vi "_VEL.vi"(0 "System no.":i32=1 min=1 max=4 step=1, 2 "Axes to set":string[](array[string]), 3 "Velocity values":dbl[](array[numeric]) format="%.6f", 4 "No.of digits":i16=4, 5 "error in":errorcluster, 6 "Without axis ID?":bool) -> (14 "Controller error":bool, 19 "error out":errorcluster)   [LabVIEW 2015]
doc: "Sets velocity and checks for error. If Without axis ID? is TRUE, then Axes to set is ignored and first field of Velocity values array is used for velocity command. The velocity should not be set to 0. Number of digits is the number of digits after the decimal point in the velocity value(s) that will be sent. Controller error is TRUE if selected system reports an error code which is not 0.\n\nValid for Analog systems, C-702, C-843, C-843.PM, C-844, C-848, C-865, C-866, C-867, C-880, C-880K005, E-516, E-517, E-710, E-712, E-725, E-753, E-755, E-761, E-861, F-206, M-8X0, Mercury™. To support analog interfacing, VI must be present for E-816 also.\n\nAnalog: Without axis ID? = FALSE; Velocity unit is µm/sec\n\nC-867: Without axis ID? = FALSE. Velocity unit is mm/s. The VEL command saves the parameters in RAM only. To save the currently valid parameters to flash ROM, where they become the power-on defaults, you must run WPA.vi. Parameter changes not saved with WPA will be lost when the C-867 is powered off.\n\nC-880: Without axis ID? = FALSE, for NanoCube axes command is not valid\n\nC-880K005: VI only supported when called through PI_Multix.vi\n\nE-516: Without axis ID? = FALSE. Velocity unit is µm/s. The VEL command saves the parameters in RAM only. To save the currently valid parameters to flash ROM, where they become the power-on defaults, you must run WPA.vi. Parameter changes not saved with WPA will be lost when the E-516 is powered off.\n\nE-517: Without axis ID? = FALSE. Velocity unit is µm/s in closed-loop operation and V/s in open-loop operation. Velocity settings made with VEL are present in RAM only and will be reset to default (\"Servo Loop Slew Rate\" value) when the controller is powered down or rebooted.\n\nE-712, E-725, E-753, E-861: Without axis ID? = FALSE. Velocity unit is µm/s. Velocity settings made with VEL are present in RAM only and will be reset to default (\"Servo Loop Slew Rate\" value) when the controller is powered down or rebooted.\n\nE-710: Without axis ID? = FALSE. Velocity unit is µm/ms.\n\nE-755: Without axis ID? = FALSE. Velocity unit is µm/s. Command not available for E-755.101.\n\nE-761: Without axis ID? = FALSE. Velocity unit is µm/ms.The VEL command saves the \"Servo Loop Slew Rate\" parameter in RAM only. To save the currently valid parameter to flash ROM, where it becomes the power-on defaults, you must run WPA.vi. Parameter changes not saved with WPA will be lost when the PC is powered off or the E-761 is rebooted.\n\nE-861: Without axis ID? = FALSE. The VEL setting only takes effect when the given axis is in closed-loop operation (servo on). For open-loop operation, use OVL instead. The maximum value which can be set with the VEL command is given by the Closed-loop velocity parameter, ID 0xA (can be changed with SPA and SEP). On power-on, the current closed-loop velocity is half the maximum.\n\nF-206: F-206 platform velocity: Without axis ID? = TRUE; velocity of axes A and/or B: Without axis ID? = False; axes K,L,M: command not valid\n\nM-8X0: M-8X0 platform velocity: Without axis ID? = TRUE; velocity of axes A and/or B: Without axis ID? = False\n\nAll other systems: Without axis ID? = FALSE"
panel:
  # "Sets velocity and checks for error.  If \"Without axis ID\" is TRUE, \nthen \"Axes to set\" is ignored and first field of \"Velocity values\" \narray is used for velocity command."
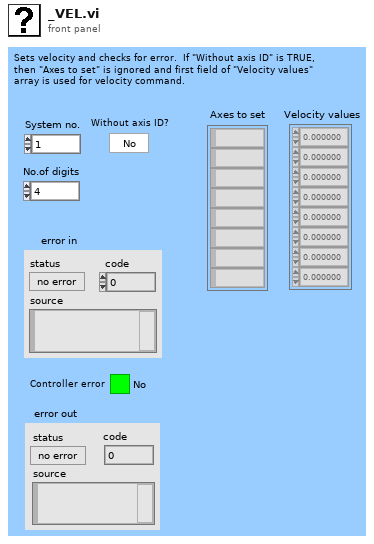
[diagram p1: front panel]
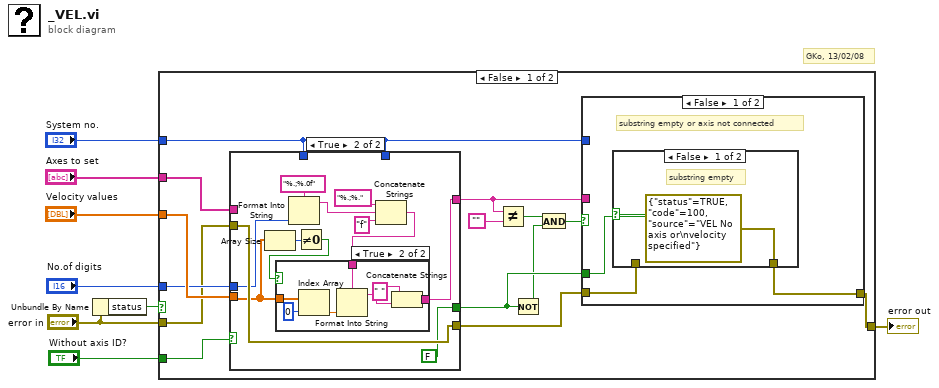
[diagram p0: block diagram]
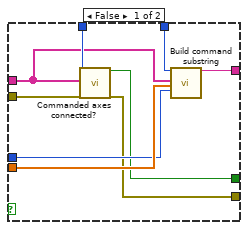
[diagram p2: hidden frame]
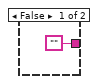
[diagram p3: hidden frame]
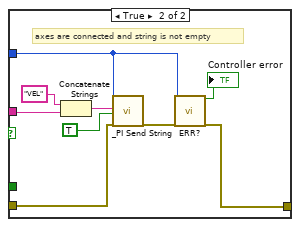
[diagram p5: hidden frame]
diagram:
  # "GKo, 13/02/08"
  n1 = Unbundle By Name("error in") -> ("status"=w2:bool)
  n2 = case shown="False" w2 {
    tunnel: [w22 w66] -> w8
    tunnel: "Velocity values" -> [w19 _]
    tunnel: "No.of digits" -> [w18 _]
    tunnel: "error in" -> [w17 w66]
    tunnel: "System no." -> [w9 _]
    tunnel: "Axes to set" -> [w15 _]
    tunnel: "Without axis ID?" -> [w10 _]
    frame False {
      n3 = case shown="True" w10 {
        tunnel: [w31 w41] -> w20
        tunnel: w19 -> [w30 w34]
        tunnel: w18 -> [w29 w36]
        tunnel: w17 -> [w28 w43]
        tunnel: [w27 w43] -> w16
        tunnel: w9 -> [w26 _]
        tunnel: w15 -> [w25 _]
        tunnel: [w24 FALSE] -> w13
        tunnel: w9 -> [w23 _]
        frame False {
          n4 = call "Commanded axes connected?.vi"("System no."=w26, "Commanded axes"=w25, "error in"=w28) -> ("Controller error"=w24:bool, "error out"=w27:errorcluster)  [unwired: 15 in]
          n5 = call "Build command substring.vi"("System no."=w23, "Affected axes"=w25, "Parameters"=w30, "No. of digits"=w29) -> ("Command substring"=w31:string)  [unwired: 15 in]
        }
        frame True {
          n6 = Array Size(array=w34) -> (size(s)=w33:i32)
          n7 = Format Into String(format string="%.;%.0f" ("Format String"), w36) -> (resulting string=w37:string)  [unwired: 2 in, 1 out]
          n8 = Not Equal To 0?(x=w33) -> (x != 0?=w32:bool)
          n9 = Concatenate Strings("%.;%." ("Format String"), w37, "f" ("Format String")) -> (w35:string)
          n10 = case shown="True" w32 {
            tunnel: ["" w47] -> w41
            tunnel: w35 -> [_ w46]
            tunnel: w34 -> [_ w45]
            frame False {
            }
            frame True {
              n11 = Index Array(array=w45, index=0 ("Index")) -> (element=w50:dbl)
              n12 = Format Into String(format string=w46, w50) -> (resulting string=w49:string)  [unwired: 2 in, 1 out]
              n13 = Concatenate Strings(" ", w49) -> (w47:string)
            }
          }
        }
      }
      n14 = Not Equal?(x=w20, y="") -> (x != y?=w14:bool)
      n15 = Not(x=w13) -> (.not. x?=w12:bool)
      n16 = And(x=w14, y=w12) -> (x .and. y?=w11:bool)
      n17 = case shown="False" w11 {
        tunnel: w20 -> [_ w64]
        tunnel: [w54 w59] -> w22
        tunnel: w16 -> [w52 w61]
        tunnel: w13 -> [w53 _]
        tunnel: w9 -> [_ w58]
        frame False {
          # "substring empty or axis not connected"
          n18 = case shown="False" w53 {
            tunnel: [errorcluster {"status"=TRUE, "code"=100, "source"="VEL No axis or\nvelocity specified"} ("error out") w56] -> w54
            tunnel: w52 -> [_ w56]
            frame False {
              # "substring empty"
            }
            frame True {
              # "commanded axis not connected"
            }
          }
        }
        frame True {
          # "axes are connected and string is not empty"
          n19 = Concatenate Strings("VEL", w64) -> (w62:string)
          n20 = call "_PI Send String.vi"("System no."=w58, "String to send"=w62, "Attach termination char.?"=TRUE ("Attach Linefeed?"), "error in"=w61) -> ("error out"=w60:errorcluster)  [unwired: 15 in]
          n21 = call "ERR?.vi"("System no."=w58, "error in"=w60) -> ("Controller error"=→"Controller error":bool, "error out"=w59:errorcluster)  [unwired: 16 in]
        }
      }
    }
    frame True {
    }
  }
  "error out" <- w8
